vi "Rename_Destination.vi"(7 "new name":string, 8 "error in (no error)":errorcluster, 9 "destTag":string, 10 "destinations in":refnum<class "IB_Destination.lvclass">[](array[class]), 11 "IB_DestTree in":refnum<class "IB_Tree_Dest.lvclass">) -> (0 "error out":errorcluster, 1 "duplicate?":bool, 2 "destinations out":refnum<class "IB_Destination.lvclass">[](array[class]), 3 "IB_DestTree out":refnum<class "IB_Tree_Dest.lvclass">, 5 "edits":T1[](array[typedef]))   [LabVIEW 2020, in "IB_Tree_Dest.lvclass"]
uses:
  <vilib>/AppBuilder/IB_Classes/Tree_Dest/IB_Tree_Dest.lvclass
  <vilib>/AppBuilder/IB_Classes/Tree_Dest/IB_Tree_Dest.lvclass/IB_Tree_Dest.ctl
  <vilib>/AppBuilder/IB_Classes/Tree/IB_Tree.lvclass
  <vilib>/AppBuilder/IB_Classes/Destination/IB_Destination.lvclass
  <vilib>/AppBuilder/IB_Classes/Tree_Dest/destEdits_operation.ctl
  <vilib>/AppBuilder/IB_Classes/Tree_Dest/destEdits_edit.ctl
  <vilib>/AppBuilder/IB_Classes/Tree_Dest/destEdits_rename.ctl
  e:/builds/penguin/labview/branches/2020/dev/dist/vi.lib/AppBuilder/IB_Classes/Tree/IB_Tree.lvclass
  e:/builds/penguin/labview/branches/2020/dev/dist/vi.lib/AppBuilder/IB_Classes/Tree_Dest/IB_Tree_Dest.lvclass
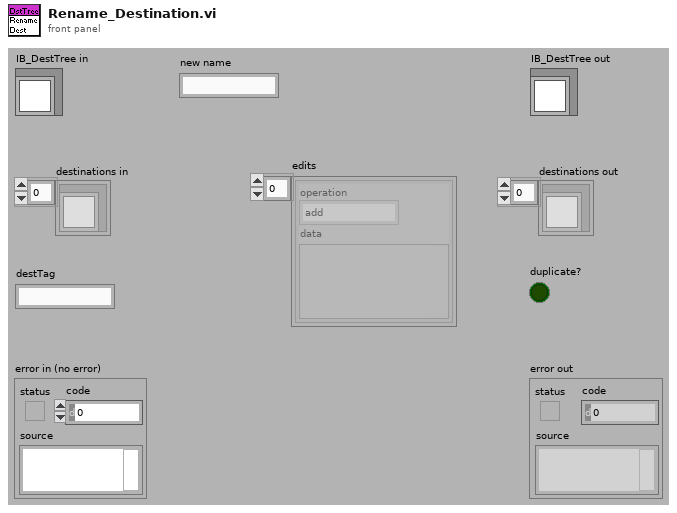
[diagram p1: front panel]
types:
  T1 = typedef "destEdits_edit.ctl" = cluster{"operation":T2, "data":variant}
  T2 = typedef "destEdits_operation.ctl" = enum16{"add", "remove", "rename", "sort children", "default dir changed"}
  T3 = typedef "destEdits_rename.ctl" = cluster{"child tag":string, "left cell string":string}
  T4 = typedef "IB_Destination.ctl" = cluster{"name":string, "unlock":bool, "parentTag":string, "destTag":string, "eng_installPath":string}
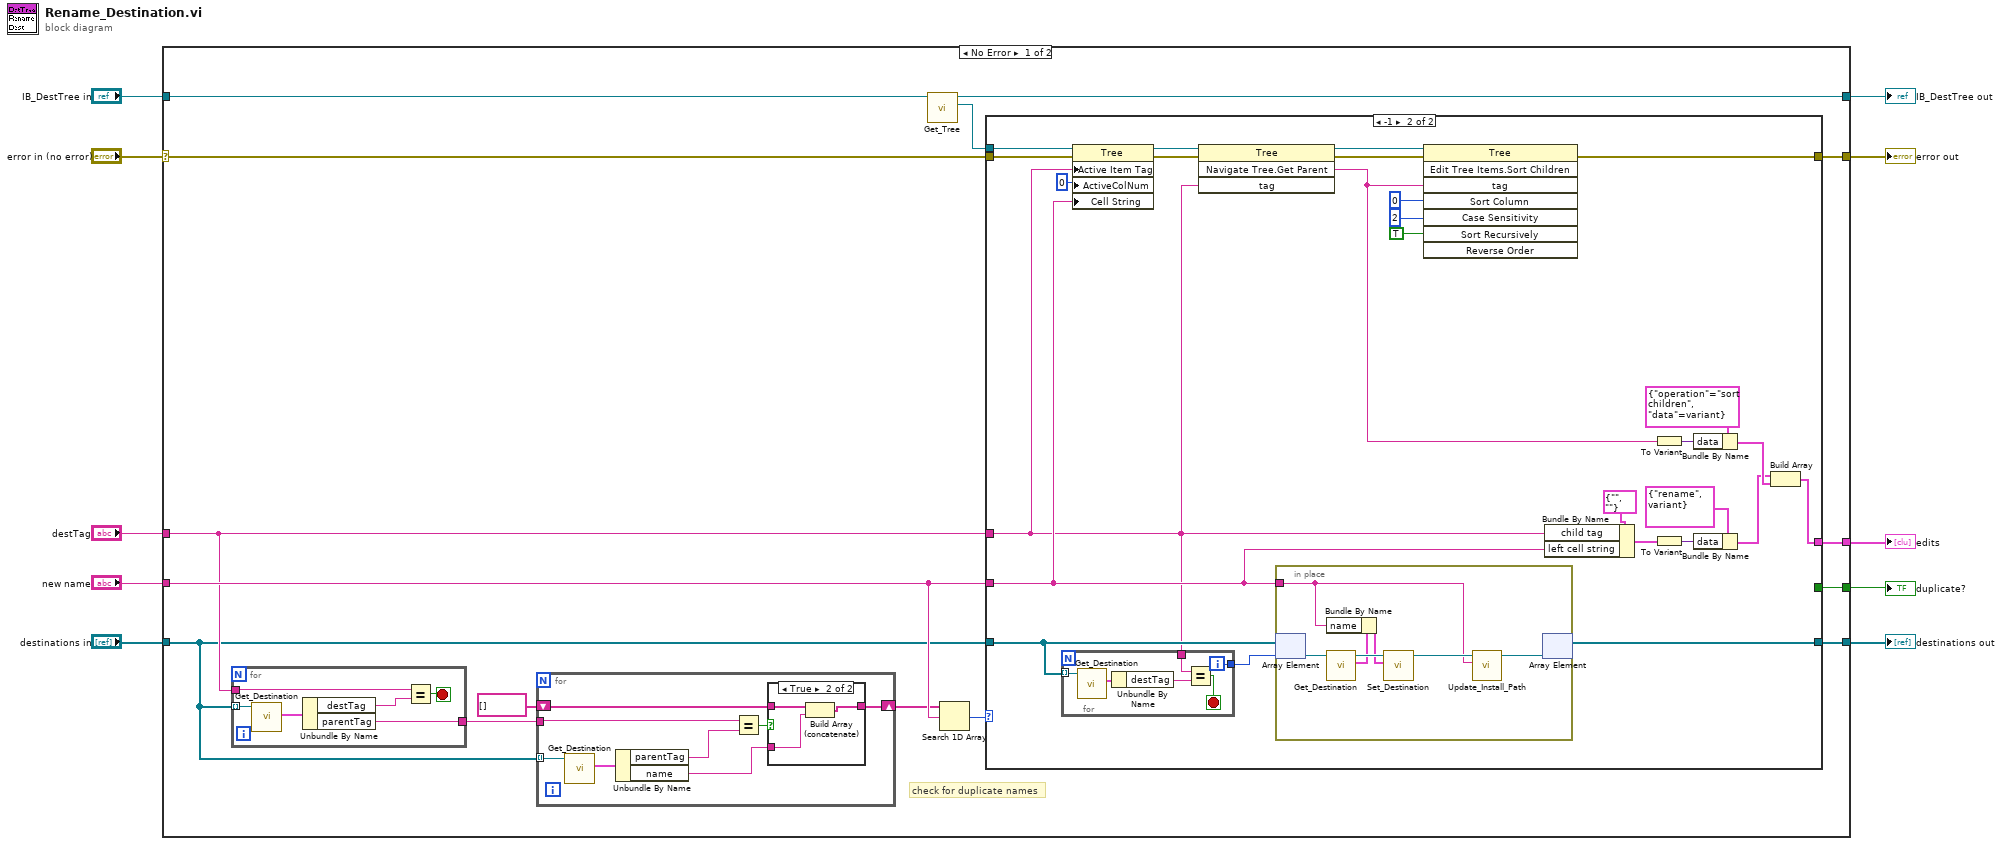
[diagram p0: block diagram]
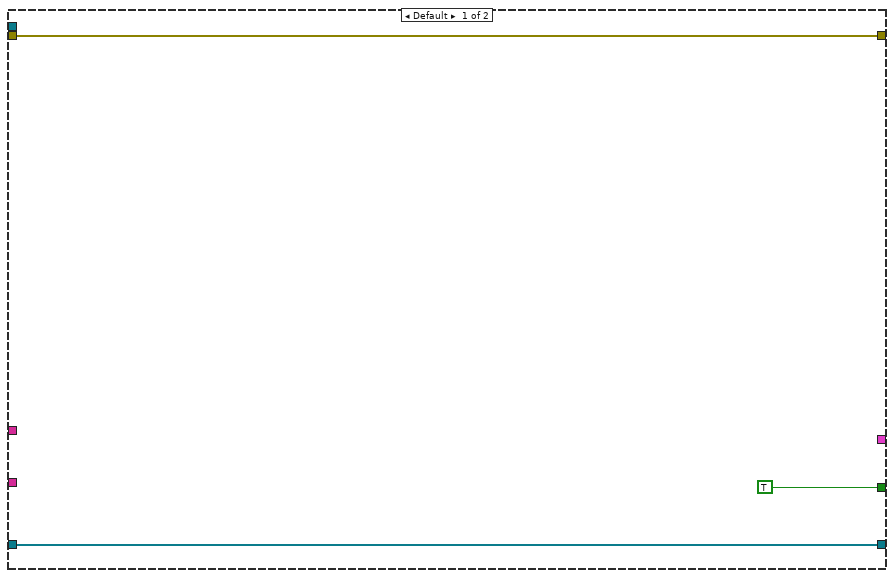
[diagram p3: hidden frame]
diagram:
  n1 = case shown="No Error" "error in (no error)" {
    selector: "error in (no error)" -> [w13 w88]
    tunnel: [w23 w88] -> w9
    tunnel: [w24 w87] -> w7
    tunnel: "IB_DestTree in" -> [w25 w87]
    tunnel: "destTag" -> [w17 _]
    tunnel: "new name" -> [w20 _]
    tunnel: "destinations in" -> [w15 w86]
    tunnel: [w21 _] -> w1
    tunnel: [w19 w86] -> w3
    tunnel: [w18 _] -> w2
    frame No Error {
      # "check for duplicate names"
      n2 = for {
        tunnel: w15 -> [w43] mode=indexing
        tunnel: w17 -> [w40]
        tunnel: [w38] -> w11
        stop <- w39 stop-if-true
        n3 = call <vilib>:"Get_Destination.vi"("IB_Destination in"=w43) -> ("data"=w42:T4)  [unwired: 1 in, 9 out]
        n4 = Unbundle By Name(w42) -> ("destTag"=w41:string, "parentTag"=w38:string)
        n5 = Equal?(x=w40, y=w41) -> (x = y?=w39:bool)
      }
      n6 = for {
        tunnel: w15 -> [w33] mode=indexing
        tunnel: w11 -> [w30]
        shift-right: [w27] -> w14
        shift-left: string[] [] -> [w29]
        n7 = call <vilib>:"Get_Destination.vi"("IB_Destination in"=w33) -> ("data"=w32:T4)  [unwired: 1 in, 9 out]
        n8 = Unbundle By Name(w32) -> ("parentTag"=w31:string, "name"=w26:string)
        n9 = Equal?(x=w30, y=w31) -> (x = y?=w28:bool)
        n10 = case shown="True" w28 {
          tunnel: w29 -> [w34 w37]
          tunnel: [w34 w36] -> w27
          tunnel: w26 -> [_ w35]
          frame False {
          }
          frame True {
            n11 = Build Array (concatenate)(w37, w35) -> (w36:string[])
          }
        }
      }
      n12 = call <vilib>:"Get_Tree.vi"("IB_Tree in"=w25) -> ("ctl"=w12:refnum<vi>, "IB_Tree out"=w24:refnum<class "IB_Tree_Dest.lvclass">)  [unwired: 1 in, 8 out]
      n13 = Search 1D Array(1D array=w14, element=w20) -> (index of element=w22:i32)  [unwired: 1 out]
      n14 = case shown="-1" w22 {
        tunnel: [w46 w62] -> w23
        tunnel: w13 -> [w46 w71]
        tunnel: w12 -> [_ w70]
        tunnel: w17 -> [_ w55]
        tunnel: w20 -> [_ w64]
        tunnel: w15 -> [w45 w69]
        tunnel: [_ w47] -> w21
        tunnel: [w45 w56] -> w19
        tunnel: [TRUE _] -> w18
        frame Default {
        }
        frame -1 {
          n15 = for {
            tunnel: w69 -> [w85] mode=indexing
            tunnel: w55 -> [w82]
            tunnel: [w80] -> w63
            i -> [w80]
            stop <- w81 stop-if-true
            n16 = call <vilib>:"Get_Destination.vi"("IB_Destination in"=w85) -> ("data"=w84:T4)  [unwired: 1 in, 9 out]
            n17 = Unbundle By Name(w84) -> ("destTag"=w83:string)
            n18 = Equal?(x=w82, y=w83) -> (x = y?=w81:bool)
          }
          n19 = property class="Tree"(reference=w70, error in=w71, "Active Item Tag"=w55, "ActiveColNum"=0 ("Active Cell:Active Column Number"), "Cell String"=w64) -> (reference out=w60:refnum<vi>, error out=w59:errorcluster)
          n20 = invoke class="Tree" method="Navigate Tree.Get Parent"(reference=w60, error in=w59, "tag"=w55) -> (reference out=w57:refnum<vi>, error out=w58:errorcluster, "Navigate Tree:Get Parent"=w50:string)  [unwired: 1 in, 1 out]
          n21 = in-place {
            in-place-border: w64 -> [w73]
            n22 = in-place-array #1(w69, w63) -> (w78:refnum<class "IB_Destination.lvclass">)
            n23 = call <vilib>:"Get_Destination.vi"("IB_Destination in"=w78) -> ("data"=w75:T4, "IB_Destination out"=w77:refnum<class "IB_Destination.lvclass">)  [unwired: 1 in, 8 out]
            n24 = Bundle By Name(cluster=w75, "name"=w73) -> (w74:T4)
            n25 = call <vilib>:"Set_Destination.vi"("data"=w74, "IB_Destination in"=w77) -> ("IB_Destination out"=w76:refnum<class "IB_Destination.lvclass">)  [unwired: 1 in, 8 out]
            n26 = call-dynamic "Update_Install_Path.vi"("destName"=w73, "IB_Destination in"=w76) -> ("IB_Destination out"=w79:refnum<class "IB_Destination.lvclass">)  [unwired: 1 in, 8 out]
            n27 = in-place-array #1(w79) -> (w56:refnum<class "IB_Destination.lvclass">[])  [unwired: 1 out]
          }
          n28 = invoke class="Tree" method="Edit Tree Items.Sort Children"(reference=w57, error in=w58, "tag"=w50, "Sort Column"=0, "Case Sensitivity"=2, "Sort Recursively"=TRUE ("Carry Children?")) -> (error out=w62:errorcluster)  [unwired: 2 in, 7 out]
          n29 = Bundle By Name(cluster=T3 {"child tag"="", "left cell string"=""} ("rename"), "child tag"=w55, "left cell string"=w64) -> (w68:T3)
          n30 = To Variant(anything=w50) -> (Variant=w51:variant)
          n31 = To Variant(anything=w68) -> (Variant=w67:variant)
          n32 = Bundle By Name(cluster=T1 {"operation"=enum."sort children", "data"=variant} ("edit"), "data"=w51) -> (w49:T1)
          n33 = Bundle By Name(cluster=T1 {"operation"=enum."rename", "data"=variant} ("edit"), "data"=w67) -> (w48:T1)
          n34 = Build Array(w48, w49) -> (w47:T1[])
        }
      }
    }
    frame Error {
    }
  }
  "error out" <- w9
  "IB_DestTree out" <- w7
  "destinations out" <- w3
  "duplicate?" <- w2
  "edits" <- w1
